vi "HELLO.vi"(4 "client name":string, 6 "AUTH":cluster{"username":string, "password":string}, 8 "error in (no error)":errorcluster, 10 "protocol version":string="3", 11 "Redis Client in":refnum<class "Redis Client.lvclass">) -> (0 "error out":errorcluster, 1 "server properties":variant, 3 "Redis Client out":refnum<class "Redis Client.lvclass">)   [LabVIEW 2019, in "Redis Client for LabVIEW.lvlib" / "Redis Client.lvclass"]
uses:
  Redis Client.lvclass
  lib/RESP3-for-LabVIEW/RESP3/subVIs/RESP3 Make String Base.vi
  lib/RESP3-for-LabVIEW/RESP3/types/RESP3 data type attribute.vi
  lib/RESP3-for-LabVIEW/RESP3/high-level/RESP3 Make Array.vi
  lib/RESP3-for-LabVIEW/RESP3/high-level/RESP3 Get String.vi
  lib/RESP3-for-LabVIEW/RESP3/RESP3.lvlib
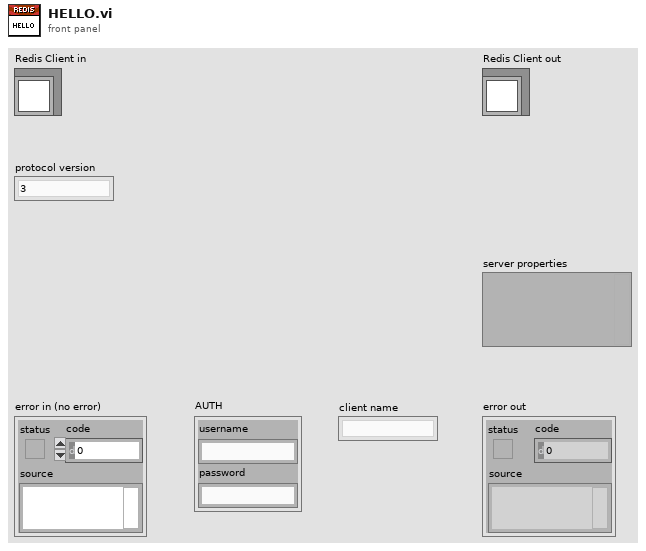
[diagram p1: front panel]
types:
  T1 = typedef "RESP3.lvlib/RESP3 Type.ctl" = enum8{"<0x00>", "<0x01>", "<0x02>", "<0x03>", "<0x04>", "<0x05>", "<0x06>", "<0x07>", "<0x08>", "<0x09>", "<0x0A>", "<0x0B>", "<0x0C>", "<0x0D>", "<0x0E>", "<0x0F>", "<0x10>", "<0x11>", "<0x12>", "<0x13>", "<0x14>", "<0x15>", "<0x16>", "<0x17>", "<0x18>", "<0x19>", "<0x1A>", "<0x1B>", "<0x1C>", "<0x1D>", "<0x1E>", "<0x1F>", "\" \"", "BLOB ERROR", "\"\"\"", "BOOLEAN", "BLOB", "MAP", "\"&\"", "\"'\"", "BIG NUMBER", "\")\"", "ARRAY", "STRING", "DOUBLE", "ERROR", "END", "\"/\"", "\"0\"", "\"1\"", "\"2\"", "\"3\"", "\"4\"", "\"5\"", "\"6\"", "\"7\"", "\"8\"", "\"9\"", "INTEGER", "STREAM", "\"<\"", "VERBATIM STRING", "PUSH", "\"?\"", "\"@\"", "\"A\"", "\"B\"", "\"C\"", "\"D\"", "\"E\"", "\"F\"", "\"G\"", "\"H\"", "\"I\"", "\"J\"", "\"K\"", "\"L\"", "\"M\"", "\"N\"", "\"O\"", "\"P\"", "\"Q\"", "\"R\"", "\"S\"", "\"T\"", "\"U\"", "\"V\"", "\"W\"", "\"X\"", "\"Y\"", "\"Z\"", "\"[\"", "\"\\\"", "\"]\"", "\"^\"", "NULL", "\"`\"", "\"a\"", "\"b\"", "\"c\"", "\"d\"", "\"e\"", "\"f\"", "\"g\"", "\"h\"", "\"i\"", "\"j\"", "\"k\"", "\"l\"", "\"m\"", "\"n\"", "\"o\"", "\"p\"", "\"q\"", "\"r\"", "\"s\"", "\"t\"", "\"u\"", "\"v\"", "\"w\"", "\"x\"", "\"y\"", "\"z\"", "\"{\"", "ATTRIBUTES", "\"}\"", "SET", "<0x7F>", "<0x80>", "<0x81>", "<0x82>", "<0x83>", "<0x84>", "<0x85>", "<0x86>", "<0x87>", "<0x88>", "<0x89>", "<0x8A>", "<0x8B>", "<0x8C>", "<0x8D>", "<0x8E>", "<0x8F>", "<0x90>", "<0x91>", "<0x92>", "<0x93>", "<0x94>", "<0x95>", "<0x96>", "<0x97>", "<0x98>", "<0x99>", "<0x9A>", "<0x9B>", "<0x9C>", "<0x9D>", "<0x9E>", "<0x9F>", "<0xA0>", "<0xA1>", "<0xA2>", "<0xA3>", "<0xA4>", "<0xA5>", "<0xA6>", "<0xA7>", "<0xA8>", "<0xA9>", "<0xAA>", "<0xAB>", "<0xAC>", "<0xAD>", "<0xAE>", "<0xAF>", "<0xB0>", "<0xB1>", "<0xB2>", "<0xB3>", "<0xB4>", "<0xB5>", "<0xB6>", "<0xB7>", "<0xB8>", "<0xB9>", "<0xBA>", "<0xBB>", "<0xBC>", "<0xBD>", "<0xBE>", "<0xBF>", "<0xC0>", "<0xC1>", "<0xC2>", "<0xC3>", "<0xC4>", "<0xC5>", "<0xC6>", "<0xC7>", "<0xC8>", "<0xC9>", "<0xCA>", "<0xCB>", "<0xCC>", "<0xCD>", "<0xCE>", "<0xCF>", "<0xD0>", "<0xD1>", "<0xD2>", "<0xD3>", "<0xD4>", "<0xD5>", "<0xD6>", "<0xD7>", "<0xD8>", "<0xD9>", "<0xDA>", "<0xDB>", "<0xDC>", "<0xDD>", "<0xDE>", "<0xDF>", "<0xE0>", "<0xE1>", "<0xE2>", "<0xE3>", "<0xE4>", "<0xE5>", "<0xE6>", "<0xE7>", "<0xE8>", "<0xE9>", "<0xEA>", "<0xEB>", "<0xEC>", "<0xED>", "<0xEE>", "<0xEF>", "<0xF0>", "<0xF1>", "<0xF2>", "<0xF3>", "<0xF4>", "<0xF5>", "<0xF6>", "<0xF7>", "<0xF8>", "<0xF9>", "<0xFA>", "<0xFB>", "<0xFC>", "<0xFD>", "<0xFE>"}
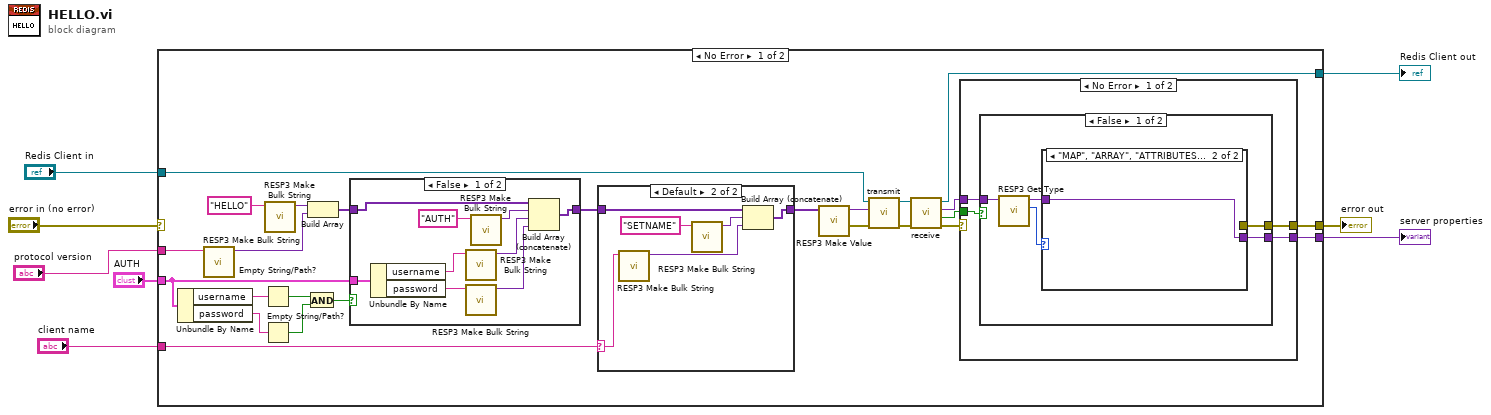
[diagram p0: block diagram]
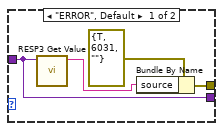
[diagram p4: hidden frame]
diagram:
  n1 = case shown="No Error" "error in (no error)" {
    selector: "error in (no error)" -> [_ w67]
    tunnel: [w30 w67] -> w7
    tunnel: "Redis Client in" -> [w33 w66]
    tunnel: [w32 w66] -> w5
    tunnel: [w31 _] -> w1
    tunnel: "protocol version" -> [w20 _]
    tunnel: "AUTH" -> [w13 _]
    tunnel: "client name" -> [w11 _]
    frame No Error {
      n2 = Unbundle By Name(w13) -> ("username"=w18:string, "password"=w17:string)
      n3 = call "RESP3 Make Bulk String.vi"("String"=w20) -> ("RESP3 Value out"=w19:variant)  [unwired: 9 in, 1 out]
      n4 = Empty String/Path?(string/path=w18) -> (empty?=w16:bool)
      n5 = Empty String/Path?(string/path=w17) -> (empty?=w15:bool)
      n6 = call "RESP3 Make Bulk String.vi"("String"="HELLO" ("string in")) -> ("RESP3 Value out"=w21:variant)  [unwired: 9 in, 1 out]
      n7 = And(x=w16, y=w15) -> (x .and. y?=w14:bool)
      n8 = Build Array(w21, w19) -> (w12:variant[])
      n9 = case shown="False" w14 {
        tunnel: w13 -> [w49 _]
        tunnel: w12 -> [w42 w50]
        tunnel: [w41 w50] -> w9
        frame False {
          n10 = Unbundle By Name(w49) -> ("username"=w47:string, "password"=w48:string)
          n11 = call "RESP3 Make Bulk String.vi"("String"=w47) -> ("RESP3 Value out"=w44:variant)  [unwired: 9 in, 1 out]
          n12 = call "RESP3 Make Bulk String.vi"("String"=w48) -> ("RESP3 Value out"=w43:variant)  [unwired: 9 in, 1 out]
          n13 = call "RESP3 Make Bulk String.vi"("String"="AUTH") -> ("RESP3 Value out"=w45:variant)  [unwired: 9 in, 1 out]
          n14 = Build Array (concatenate)(w42, w45, w44, w43) -> (w41:variant[])
        }
        frame True {
        }
      }
      n15 = case shown="Default" w11 {
        selector: w11 -> [_ w37]
        tunnel: [w34 w35] -> w10
        tunnel: w9 -> [w34 w36]
        frame "" {
        }
        frame Default {
          n16 = call "RESP3 Make Bulk String.vi"("String"=w37) -> ("RESP3 Value out"=w38:variant)  [unwired: 9 in, 1 out]
          n17 = call "RESP3 Make Bulk String.vi"("String"="SETNAME") -> ("RESP3 Value out"=w39:variant)  [unwired: 9 in, 1 out]
          n18 = Build Array (concatenate)(w36, w39, w38) -> (w35:variant[])
        }
      }
      n19 = call-poly "RESP3 Make Value.vi"("RESP3 Values in"=w10) -> ("error out"=w24:errorcluster, "RESP3 Value out"=w23:variant)  [unwired: 9 in]
      n20 = call-dynamic "transmit.vi"("error in (no error)"=w24, "RESP3 Value"=w23, "Redis Client in"=w33) -> ("error out"=w28:errorcluster, "Redis Client out"=w29:refnum<class "Redis Client.lvclass">)  [unwired: 7 in]
      n21 = call-dynamic "receive.vi"("error in (no error)"=w28, "Redis Client in"=w29) -> ("error out"=w25:errorcluster, "timed out?"=w26:bool, "RESP3 Value"=w27:variant, "Redis Client out"=w32:refnum<class "Redis Client.lvclass">)  [unwired: 6 in]
      n22 = case shown="No Error" w25 {
        selector: w25 -> [_ w65]
        tunnel: [w54 _] -> w31
        tunnel: [w53 w65] -> w30
        tunnel: w27 -> [w52 _]
        tunnel: w26 -> [w51 _]
        frame No Error {
          n23 = case shown="False" w51 {
            tunnel: [w59 _] -> w54
            tunnel: [w58 _] -> w53
            tunnel: w52 -> [w56 _]
            frame False {
              n24 = call "RESP3 Get Type.vi"("RESP3 Value in"=w56) -> ("RESP3 Type"=w55:T1, "RESP3 Value out"=w57:variant)  [unwired: 7 in, 2 out]
              n25 = case shown="\"MAP\", \"ARRAY\", \"ATTRIBUTES\"" w55 {
                tunnel: [w60 w64] -> w59
                tunnel: [w61 _] -> w58
                tunnel: w57 -> [w60 w64]
                frame "ERROR", Default {
                  n26 = call-poly "RESP3 Get Value.vi"("RESP3 Value in"=w60) -> ("String out"=w62:string)  [unwired: 7 in, 3 out]
                  n27 = Bundle By Name(cluster=errorcluster {"status"=TRUE, "code"=6031, "source"=""} ("error constant"), "source"=w62) -> (w61:errorcluster)
                }
                frame "MAP", "ARRAY", "ATTRIBUTES" {
                }
              }
            }
            frame True {
            }
          }
        }
        frame Error {
        }
      }
    }
    frame Error {
    }
  }
  "error out" <- w7
  "Redis Client out" <- w5
  "server properties" <- w1
